vi "Client PC - Test Outbound Traffic from Server.vi"(8 "error in (no error)":errorcluster, 11 "ports to check":u16[](array[numeric])=[82, 482, 5672, 6343, 8002, 49580, 3580, 80, 22, 44516, 52725, 8080]) -> (0 "error out":errorcluster, 2 "log file path":path, 3 "Results":string[][](array[string]))   [LabVIEW 2019]
doc: "Demonstrates how to open a connection to an TCP server, read the data being sent, and display the data on a chart. This VI is designed to stop if the TCP connection is terminated."
panel:
  out "log file name":string
  out "current test":cluster{string, "error out":errorcluster}
  in  "Start test":bool
  out "current port":u16
  in  "server address":string="localhost"
  out "Waveform Graph":dbl[](graph)
  # "Instructions:\n1. Ensure Test server Outbound - Server  is already running.\n2. Run this exe\n3. Click on the button Start Test \n4. Click Stop to stop the VI. Note that if you stop the server VI, this VI will stop automatically."
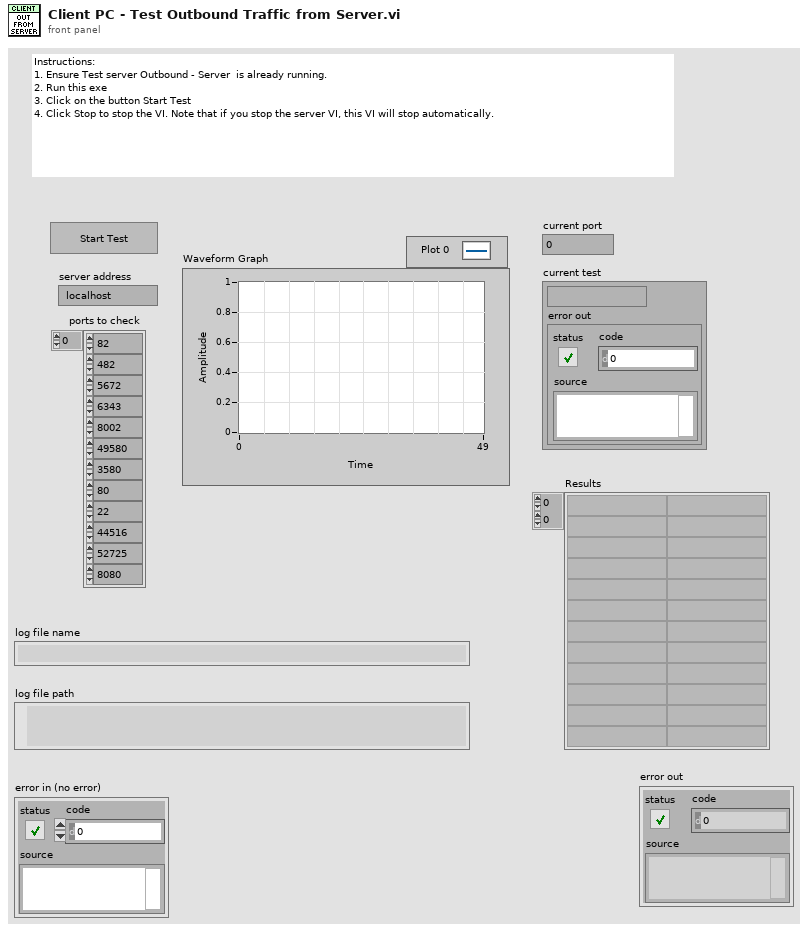
[diagram p1: front panel]
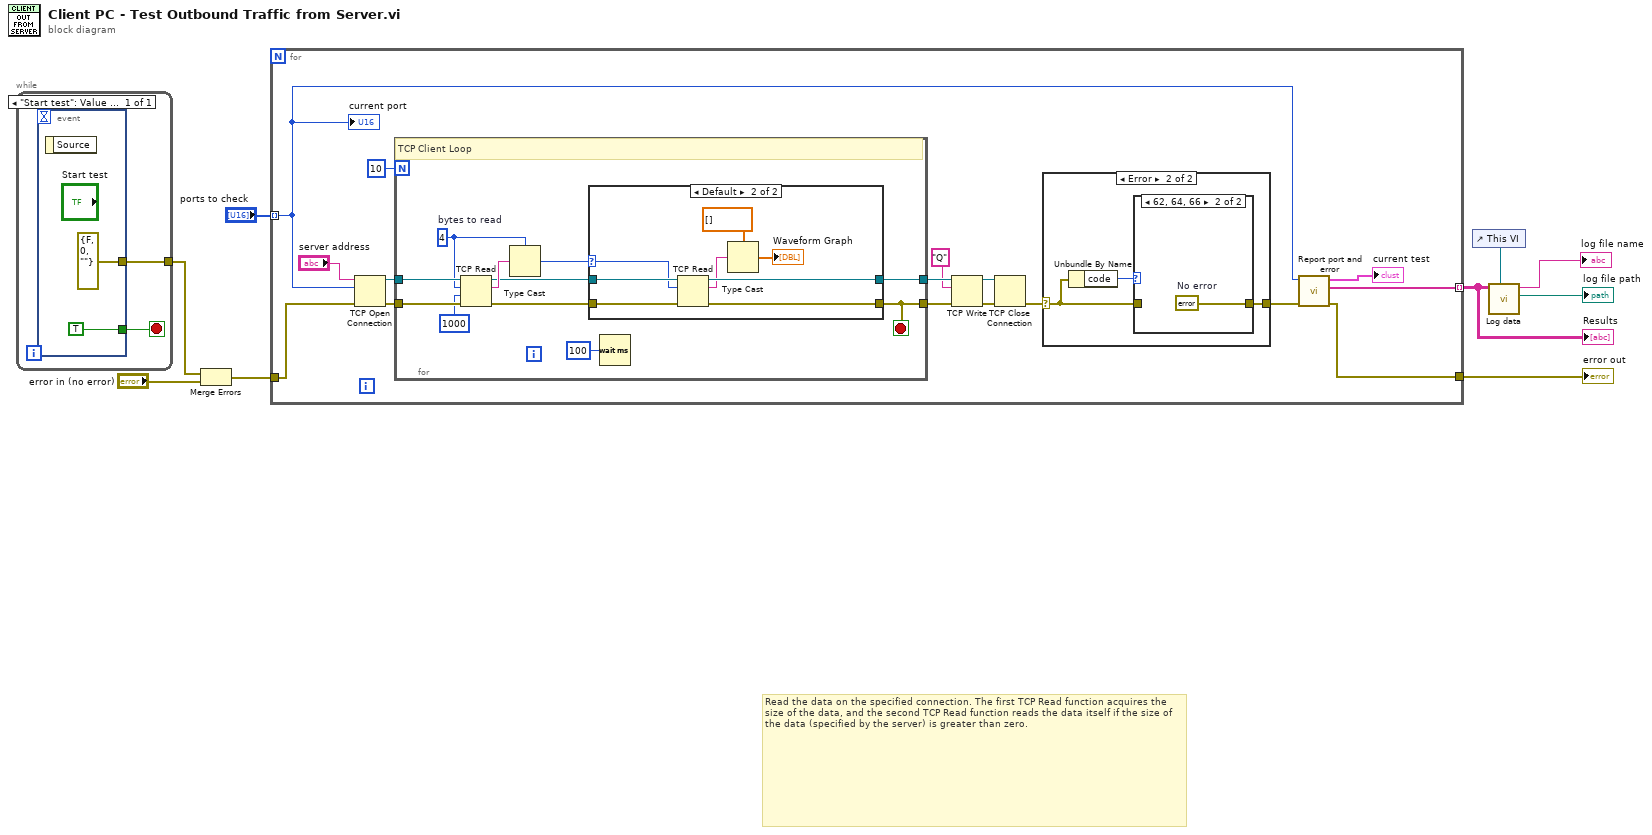
[diagram p0: block diagram]
diagram:
  # "Read the data on the specified connection. The first TCP Read function acquires the size of the data, and the second TCP Read function reads the data itself if the size of the data (specified by the server) is greater than zero."
  n1 = while {
    tunnel: [w11] -> w4
    stop <- w10 stop-if-true
    n2 = event shown="[0] \"Start test\": Value Change" {
      selector: _ -> [_]
      dyn-events: _ -> [_]
      timeout: _ -> [_]
      tunnel: [errorcluster {"status"=FALSE, "code"=0, "source"=""} ("error constant")] -> w11
      tunnel: [TRUE] -> w10
      event "Start test": Value Change {
        n3 = event-data() -> ()  [unwired: 1 in, 1 out]
      }
    }
  }
  n4 = Merge Errors(w4, "error in (no error)") -> (w2:errorcluster)
  n5 = for {
    tunnel: "ports to check" -> [w16] mode=indexing
    tunnel: [w18] -> w8 mode=indexing
    tunnel: w2 -> [w14]
    tunnel: [w15] -> w1
    n6 = TCP Open Connection(address="server address", remote port or service name=w16, error in (no error)=w14) -> (connection ID=w29:refnum<k5>, error out=w28:errorcluster)  [unwired: 2 in]
    n7 = for {
      N: 10 -> [_]
      tunnel: w28 -> [w36]
      tunnel: w29 -> [w37]
      tunnel: [w33] -> w26
      tunnel: [w32] -> w24
      stop <- w32 stop-if-true
      w35 = 4  # bytes to read
      # "TCP Client Loop"
      n8 = TCP Read(connection ID=w37, bytes to read=w35, error in (no error)=w36, 9:1000 ("timeout ms (25000)")) -> (connection ID out=w39:refnum<k5>, data out=w40:string, error out=w38:errorcluster)  [unwired: 1 in]
      n9 = Type Cast(type=w35, x=w40) -> (*(type *) &x=w31:i32)
      n10 = case shown="Default" w31 {
        selector: w31 -> [_ w43]
        tunnel: w39 -> [w42 w50]
        tunnel: w38 -> [w41 w49]
        tunnel: [w42 w46] -> w33
        tunnel: [w41 w45] -> w32
        frame ..0 {
          # "The server has not written any data"
        }
        frame Default {
          n11 = TCP Read(connection ID=w50, bytes to read=w43, error in (no error)=w49) -> (connection ID out=w46:refnum<k5>, data out=w44:string, error out=w45:errorcluster)  [unwired: 2 in]
          n12 = Type Cast(type=dbl[] [] ("chart"), x=w44) -> (*(type *) &x=→"Waveform Graph":dbl[])
        }
      }
      n13 = Wait (ms)(milliseconds to wait=u32 100) -> ()  [unwired: 1 out]
    }
    n14 = TCP Write(connection ID=w26, data in="Q", error in (no error)=w24) -> (connection ID out=w27:refnum<k5>, error out=w25:errorcluster)  [unwired: 2 out]
    n15 = TCP Close Connection(connection ID=w27, error in (no error)=w25) -> (error out=w22:errorcluster)  [unwired: 1 in, 1 out]
    n16 = case shown="Error" w22 {
      selector: w22 -> [w51 w53]
      tunnel: [w51 w52] -> w19
      frame No Error {
      }
      frame Error {
        n17 = Unbundle By Name(w53) -> ("code"=w54:i32)
        n18 = case shown="62, 64, 66" w54 {
          tunnel: w53 -> [w55 _]
          tunnel: [w55 w56] -> w52
          frame Default {
          }
          frame 62, 64, 66 {
            w56 = errorcluster {"status"=FALSE, "code"=0, "source"=""}  # No error
          }
        }
      }
    }
    n19 = call "Report port and error.vi"("error in (no error)"=w19, "port"=w16) -> ("error out"=w15:errorcluster, "Array"=w18:string[], "output cluster"=→"current test":cluster{string, "error out":errorcluster})  [unwired: 7 in]
    "current port" <- w16
  }
  "Results" <- w8
  "error out" <- w1
  n20 = control-ref of="This VI"() -> (w5:refnum<vi>)
  n21 = call "Log data.vi"(7:w5, 11:w8) -> ("log file path"=→"log file path":path, "log file name"=→"log file name":string)  [unwired: 7 in, 1 out]
